vi "array3.vi"() -> ()   [LabVIEW 2019]
panel:
  out "ans":dbl
  in  "b":dbl
  in  "a":dbl
  in  "stop":bool
  out "arr":bool[](array[boolean])
  in  "/":bool
  in  "*":bool
  in  "-":bool
  in  "+":bool
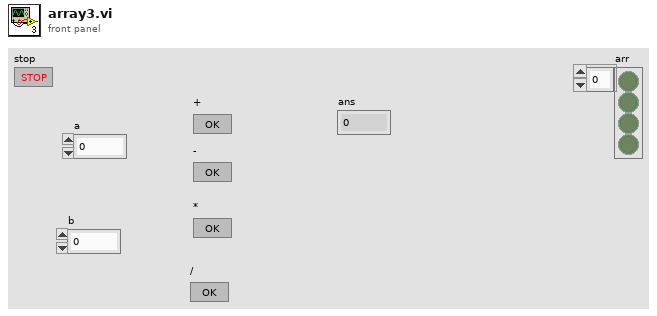
[diagram p1: front panel]
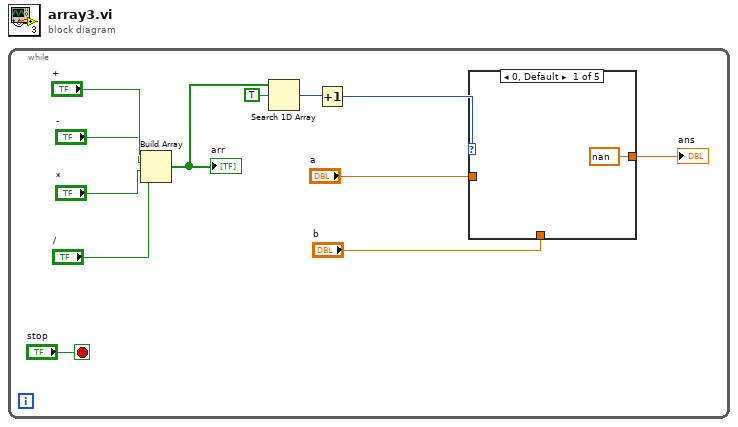
[diagram p0: block diagram]
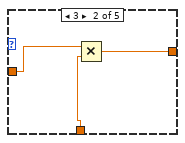
[diagram p2: hidden frame]
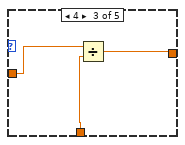
[diagram p3: hidden frame]
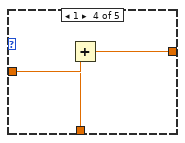
[diagram p4: hidden frame]
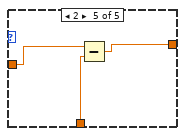
[diagram p5: hidden frame]
diagram:
  n1 = while {
    stop <- "stop" stop-if-true
    n2 = Build Array("+", "-", "*", "/") -> (w8:bool[])
    "arr" <- w8
    n3 = Search 1D Array(1D array=w8, element=TRUE) -> (index of element=w5:i32)  [unwired: 1 in]
    n4 = Increment(x=w5) -> (x+1=w4:i32)
    n5 = case shown="0, Default" w4 {
      tunnel: "a" -> [_ w16 w19 w22 w25]
      tunnel: "b" -> [_ w15 w18 w21 w24]
      tunnel: [nan w14 w17 w20 w23] -> w1
      frame 0, Default {
      }
      frame 3 {
        n6 = Multiply(x=w16, y=w15) -> (x*y=w14:dbl)
      }
      frame 4 {
        n7 = Divide(x=w19, y=w18) -> (x/y=w17:dbl)
      }
      frame 1 {
        n8 = Add(x=w22, y=w21) -> (x+y=w20:dbl)
      }
      frame 2 {
        n9 = Subtract(x=w25, y=w24) -> (x-y=w23:dbl)
      }
    }
    "ans" <- w1
  }
